vi "Distance Drive Mode.vi"(0 "Y Output High":dbl, 1 "Y Output Low":dbl, 5 "Y target":dbl, 9 "Heading target":dbl, 12 "Reinitialize":bool) -> (4 "isFinished":bool, 6 "Y out":dbl, 14 "Dist Drive Status":T1, 15 "X out":dbl)   [LabVIEW 2015]
uses:
  Common Code/Dist Drive Status.ctl
  Common Code/Drivetrain Output Range.ctl
  Common Code/Change Detect Double.vi
  Robot Global Data.vi
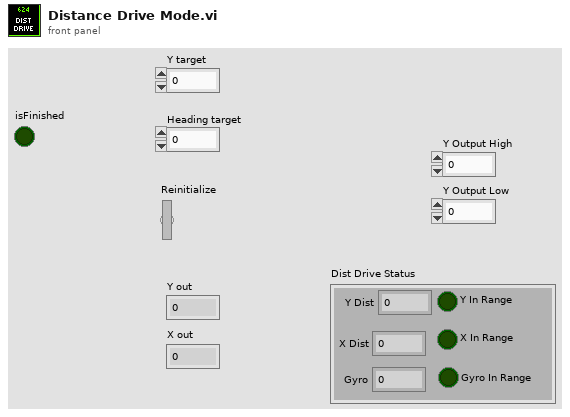
[diagram p1: front panel]
types:
  T1 = typedef "Dist Drive Status.ctl" = cluster{"Y In Range":bool, "X In Range":bool, "Gyro In Range":bool, "Y Dist":dbl, "X Dist":dbl, "Gyro":dbl}
  T2 = typedef "Drivetrain Output Range.ctl" = cluster{"output high":dbl, "output low":dbl}
  T3 = typedef "Dashboard Control Data.ctl" = cluster{"Shooter Presets":T4, "Encoder Control":T6, "Steer PID output":cluster{"output high":dbl, "output low":dbl}, " Steer PID gains":cluster{"proportional gain (Kc)":dbl, "integral time (Ti, min)":dbl, "derivative time (Td, min)":dbl}, "Drivetrain Settings":T7, "Vision Packet":T8, "Dashboard Drivetrain Command":T9, "Info/Command Cluster":T11, "Ball Vision Packet":T12, "Intake Presets":T14}
  T4 = typedef "Shooter Presets.ctl" = cluster{"Batter Shot":T5, "Low Bar Curve Shot":T5, "Deep Middle Shot":T5, "Manual Shot":T5, "Left Ticks Per Rotation":dbl, "Right Ticks Per Rotation":dbl, "Low Bar Shot":T5, "Shooter RPM Tolerance":dbl, "IIR Filter Power":dbl, "Trigger Power":dbl, "Fire from Load Delay":i32, "Angle Pot Scale Factor":dbl, "Angle Pot Zero":dbl, "Shooter Deck Length":dbl, "String Pot Dist From Pivot":dbl, "Angle PID gains":cluster{"proportional gain (Kc)":dbl, "integral time (Ti, min)":dbl, "derivative time (Td, min)":dbl}, "Angle Motor Output Range":cluster{"output high":dbl, "output low":dbl}, "Shooter Angle Tolerance":dbl, "Vision Shoot m":dbl, "Vision Shoot b":dbl, "Dist from Axis Cam to Pivot":dbl, "High Goal Center Height":dbl, "Feed Forward Max Accel":dbl, "Feed Forward Kv":dbl, "Backwards Trigger":dbl, "Shot Finish Delay (ms)":dbl}
  T5 = typedef "Shot Presets.ctl" = cluster{"Left Wheel RPM":dbl, "Right Wheel RPM":dbl, "Angle":dbl}
  T6 = typedef "Encoder Control.ctl" = cluster{"Right Tick Constant":dbl, "Left Tick Constant":dbl, "Reset?":bool, "Y Dist":cluster{"PID gains":cluster{"proportional gain (Kc)":dbl, "integral time (Ti, min)":dbl, "derivative time (Td, min)":dbl}}, "Y Stop Thresh":dbl, "Y Stop Speed":dbl}
  T7 = typedef "Drivetrain Settings.ctl" = cluster{"Gyro Tolerance":dbl, "Throttle Ramp (ms)":dbl, "Angular rate compensation":bool, "Throttle to Rate Scale":dbl, "Rate compensation gain":dbl, "Kv":dbl, "Ka":dbl, "Feed Forward P":dbl, "Feed Forward D":dbl}
  T8 = typedef "Goal Vision Packet.ctl" = cluster{"Distance":dbl, "Center X":dbl, "Center Y":dbl, "Found Target?":bool}
  T9 = typedef "Dashboard Drivetrain Command.ctl" = cluster{"Drivetrain Vision":T10, "Vision Scale Down Speed":dbl, "Vision PID gains":cluster{"proportional gain (Kc)":dbl, "integral time (Ti, min)":dbl, "derivative time (Td, min)":dbl}}
  T10 = typedef "Drivetrain Vision.ctl" = cluster{"High parameters":dbl, "Low parameters":dbl}
  T11 = typedef "Ball Tracking Command Cluster.ctl" = cluster{"Distance to Ball":dbl, "Desired Angle":dbl, "Command":enum16{"Turn to Ball", "Turn to Angle", "Get Distance"}, "Pixels from Center":dbl}
  T12 = typedef "Ball Vision Packet.ctl" = cluster{"Ball Detected?":bool, "Distance to Ball":dbl, "Desired Angle":dbl, "Pixels from Center":dbl, "Tracking mode":T13}
  T13 = typedef "Tracking Mode.ctl" = enum16{"Turn to Ball", "Turn to Angle"}
  T14 = typedef "Intake Presets.ctl" = cluster{"Intake Speed":dbl, "Outake Speed":dbl, "Low Height":dbl, "High Height":dbl, "Full Height":dbl, "Angle Speed":dbl, "Fast Angle":dbl, "Encoder Scale Factor":dbl, "Override IR":dbl, "Load Height":dbl}
  T15 = typedef "Encoder Values Super Cluster.ctl" = cluster{"Left Encoder":T16, "Right Encoder":T16}
  T16 = typedef "Encoder Values.ctl" = cluster{"Distance":dbl, "Speed":dbl, "Ticks":dbl}
  T17 = cluster{"PID gains":cluster{"proportional gain (Kc)":dbl, "integral time (Ti, min)":dbl, "derivative time (Td, min)":dbl}}
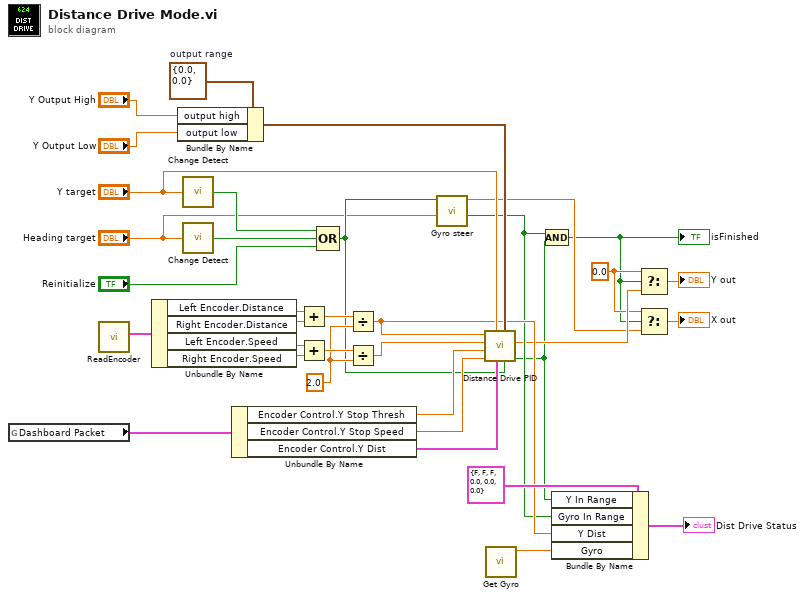
[diagram p0: block diagram]
diagram:
  w4 = 0.0 ("t")
  w17 = T2 {"output high"=0.0, "output low"=0.0}  # output range
  w25 = 2.0 ("y")
  n1 = global read "Robot Global Data.vi" "Dashboard Packet"() -> (w24:T3)
  n2 = call "ReadEncoder.vi"() -> ("Quick Use Cluster"=w22:T15)  [unwired: 11 in]
  n3 = Unbundle By Name(w22) -> ("Left Encoder.Distance"=w29:dbl, "Right Encoder.Distance"=w30:dbl, "Left Encoder.Speed"=w31:dbl, "Right Encoder.Speed"=w32:dbl)
  n4 = Bundle By Name(cluster=w17, "output high"="Y Output High", "output low"="Y Output Low") -> (w16:T2)
  n5 = call-poly "Change Detect.vi"("In"="Y target") -> ("Changed?"=w33:bool)
  n6 = call-poly "Change Detect.vi"("In"="Heading target") -> ("Changed?"=w35:bool)
  n7 = Unbundle By Name(w24) -> ("Encoder Control.Y Stop Thresh"=w21:dbl, "Encoder Control.Y Stop Speed"=w20:dbl, "Encoder Control.Y Dist"=w23:T17)
  n8 = Add(x=w29, y=w30) -> (x+y=w27:dbl)
  n9 = Add(x=w31, y=w32) -> (x+y=w28:dbl)
  n10 = Compound Arithmetic op=OR(w33, w35, "Reinitialize") -> (w14:bool)
  n11 = Divide(x=w27, y=w25) -> (x/y=w9:dbl)
  n12 = Divide(x=w28, y=w25) -> (x/y=w26:dbl)
  n13 = call "Gyro steer.vi"("Target Angle"="Heading target", "Changed?"=w14) -> ("In Range?"=w8:bool, "X out"=w3:dbl)  [unwired: 8 in]
  n14 = call "Distance Drive PID.vi"("reinitialize? (F)"=w14, "output range"=w16, "PID Params"=w23, "Setpoint"="Y target", "Max Stop Speed"=w20, "Distance Stop"=w21, "Current Speed"=w26, "Current Distance"=w9) -> ("Finished"=w1:bool, "output"=w7:dbl)  [unwired: 2 in]
  n15 = call "Get Gyro.vi"() -> ("Angle"=w10:dbl)  [unwired: 11 in]
  n16 = Compound Arithmetic op=AND(w8, w1) -> (w2:bool)
  "isFinished" <- w2
  n17 = Bundle By Name(cluster=T1 {"Y In Range"=FALSE, "X In Range"=FALSE, "Gyro In Range"=FALSE, "Y Dist"=0.0, "X Dist"=0.0, "Gyro"=0.0} ("Dist Drive Status"), "Y In Range"=w1, "Gyro In Range"=w8, "Y Dist"=w9, "Gyro"=w10) -> (→"Dist Drive Status":T1)
  n18 = Select(t=w4, s=w2, f=w7) -> (s? t:f=→"Y out":dbl)
  n19 = Select(t=w4, s=w2, f=w3) -> (s? t:f=→"X out":dbl)
